vi "JSON ReadStringsArray.vi"(8 "error in (no error)":errorcluster, 9 "Key":string, 11 "JSON":string) -> (0 "error out":errorcluster, 2 "Value":string[](array[string]))   [LabVIEW 2020, in "Error Provider API.lvlib"]
uses:
  <vilib>/NI VeriStand/Error Provider API/Error Provider API.lvlib
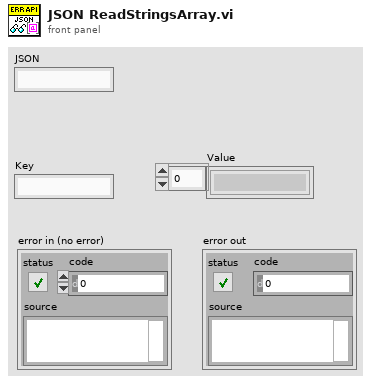
[diagram p1: front panel]
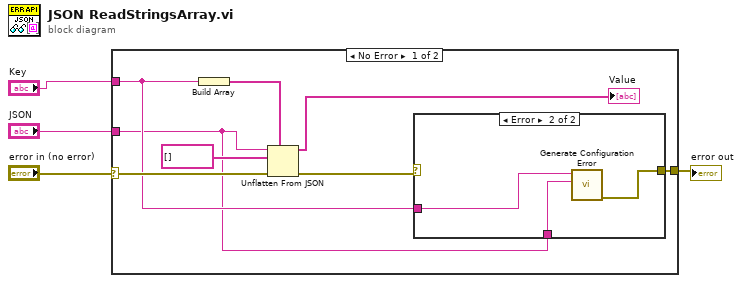
[diagram p0: block diagram]
diagram:
  n1 = case shown="No Error" "error in (no error)" {
    selector: "error in (no error)" -> [w7 w17]
    tunnel: "JSON" -> [w5 _]
    tunnel: "Key" -> [w6 _]
    tunnel: [w8 w17] -> w2
    frame No Error {
      n2 = Build Array(w6) -> (w12:string[])
      n3 = Unflatten From JSON(path=w12, JSON string=w5, type and defaults=string[] [], error in (no error)=w7) -> (value=→"Value":string[], error out=w9:errorcluster)  [unwired: 3 in]
      n4 = case shown="Error" w9 {
        selector: w9 -> [w13 _]
        tunnel: [w13 w15] -> w8
        tunnel: w6 -> [_ w16]
        tunnel: w5 -> [_ w14]
        frame No Error {
        }
        frame Error {
          n5 = call <vilib>:"Generate Configuration Error.vi"("JSON"=w14, "Key"=w16) -> ("error out"=w15:errorcluster)  [unwired: 9 in]
        }
      }
    }
    frame Error {
    }
  }
  "error out" <- w2
